vi "Time.TimeStamp to SQL DateTime String.vi"(11 "Time Stamp in":timestamp) -> (3 "Time String Out":string)   [LabVIEW 2019]
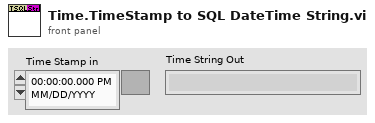
[diagram p1: front panel]
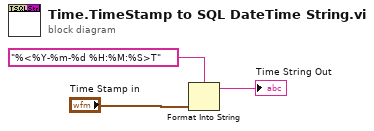
[diagram p0: block diagram]
diagram:
  n1 = Format Into String(format string="%<%Y-%m-%d %H:%M:%S>T", "Time Stamp in") -> (resulting string=→"Time String Out":string)  [unwired: 2 in, 1 out]
